vi "Memory.Pointer.Read.Safe.1D.I32.vi"(8 "error in (no error)":errorcluster, 9 "count":u64 format="%d elements", 10 "buffer in":i32[](array[numeric]), 11 "pointer in":refnum<class "Memory.Pointer.lvclass">) -> (0 "error out":errorcluster, 1 "count out":u64 format="%d elements", 2 "buffer out":i32[](array[numeric]), 3 "pointer out":refnum<class "Memory.Pointer.lvclass">)   [LabVIEW 2016, in "Memory Manager.lvlib" / "Memory.Pointer.lvclass"]
doc: "Reads from the address specified by <b>pointer</b> into <b>value</b>.\n\n<b>Note:</b> This VI is <b>safe</b>.\n\nSafe means that this function evaluates the size parameter of <b>pointer</b> to ensure that is inbounds of allocated memory before peforming a memory read/write. Reading/writing more data to a pointer than it has allocated can corrupt or crash LabVIEW."
uses:
  Memory.Pointer.lvclass
  Memory.Pointer.lvclass/Memory.Pointer.ctl
  Accessors/Get Address.vi
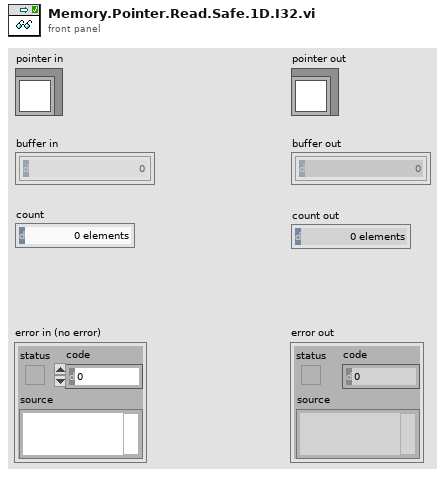
[diagram p1: front panel]
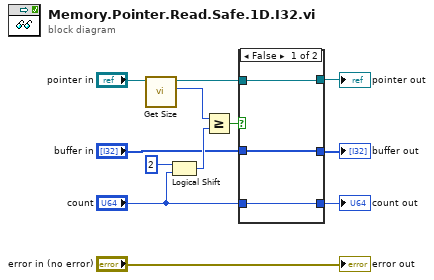
[diagram p0: block diagram]
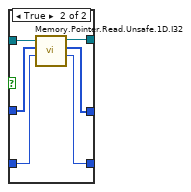
[diagram p2: hidden frame]
diagram:
  n1 = call "Get Size.vi"("Pointer in"="pointer in") -> ("size"=w9:u64, "Pointer out"=w7:refnum<class "Memory.Pointer.lvclass">)  [unwired: 8 in, 1 out]
  n2 = Logical Shift(y=i16 2, x="count") -> (x << y=w10:u64)
  n3 = Greater Or Equal?(x=w9, y=w10) -> (x >= y?=w8:bool)
  n4 = case shown="False" w8 {
    tunnel: w7 -> [w15 w21]
    tunnel: [w15 w20] -> w6
    tunnel: "buffer in" -> [w14 w19]
    tunnel: "count" -> [w13 w18]
    tunnel: [w14 w17] -> w3
    tunnel: [w13 w16] -> w2
    frame False {
    }
    frame True {
      n5 = call "Memory.Pointer.Read.Unsafe.1D.I32.vi"("count"=w18, "buffer in"=w19, "pointer in"=w21) -> ("count out"=w16:u64, "buffer out"=w17:i32[], "pointer out"=w20:refnum<class "Memory.Pointer.lvclass">)  [unwired: 5 in, 1 out]
    }
  }
  "pointer out" <- w6
  "buffer out" <- w3
  "count out" <- w2
  "error out" <- "error in (no error)"
